vi "DAG.vi"(4 "edges":cluster{"start":i32, "end":i32}[](array[cluster])) -> (0 "DAG out":refnum<class "DAG.lvclass">)   [LabVIEW 2014, in "DAG.lvclass"]
uses:
  DAG.lvclass
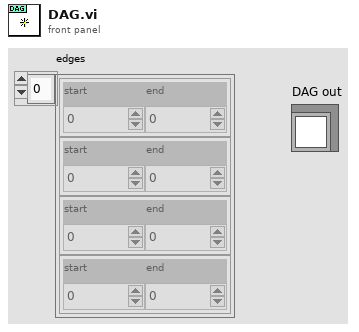
[diagram p1: front panel]
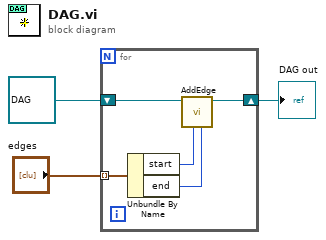
[diagram p0: block diagram]
diagram:
  n1 = for {
    shift-right: [w6] -> w1
    shift-left: refnum<class "DAG.lvclass"> refnum ("DAG out") -> [w7]
    tunnel: "edges" -> [w8] mode=indexing
    n2 = Unbundle By Name(w8) -> ("start"=w5:i32, "end"=w4:i32)
    n3 = call "AddEdge.vi"("end"=w4, "start"=w5, "DAG in"=w7) -> ("DAG out"=w6:refnum<class "DAG.lvclass">)  [unwired: 6 in]
  }
  "DAG out" <- w1
